vi "压电喷油器控制-与PLC进行串行通信完善喷油延时.vi"() -> ()   [LabVIEW 2018]
uses:
  <vilib>/Instr/_visa.llb/VISA Configure Serial Port (Instr).vi
panel:
  in  "充放电时间US":dbl[](array[numeric])=[30.0, 0.0, 70.0, 1.0, 50.0, 1.0, 0.0, 0.0, 0.0, 0.0, 0.0, 30.0]
  out "返回指令码":dbl[](array[numeric])
  in  "确定 3":bool
  in  "VISA资源名称 3":refnum<visa-resource-name>
  out "返回指令码":dbl[](array[numeric])
  in  "确定 2":bool
  in  "VISA资源名称 2":refnum<visa-resource-name>
  in  "喷油间隔设定  US":dbl[](array[numeric])=[20.0, 0.0, 0.0, 0.0, 0.0, 0.0, 0.0, 0.0, 0.0, 0.0, 0.0, 20.0]
  out "返回指令码":dbl[](array[numeric])
  in  "喷油脉宽设定 US":dbl[](array[numeric])=[10.0, 0.0, 0.0, 0.0, 0.0, 0.0, 0.0, 0.0, 0.0, 0.0, 0.0, 10.0]
  in  "允许通讯":bool
  in  "确定1":bool
  in  "VISA资源名称":refnum<visa-resource-name>
  # "每次打开上位机界面，有的数据表格可能不需要输入数据，如喷油4次，则第五个数据就不需要输入，但\n是仍然要向其写入0，相当于赋初值，否则报错。"
  # "注\n意"
  # "说明：每一行数据的第一个数据都表示指令码，其中喷油脉宽设定的指令码是10，因此第一个框中只能输入10，类似的，其余变量的指令码如下：\n喷油脉宽设定10，喷油间隔设定20，充放电时间及次数设定30"
  # "脉宽\n设定"
  # "末位校验，必须输入10"
  # "脉宽1（千百位）"
  # "脉宽1（十个位）"
  # "脉宽2（千百位）"
  # "脉宽2（十个位）"
  # "脉宽3（千百位）"
  # "脉宽3（十个位）"
  # "脉宽4（千百位）"
  # "脉宽5（千百位）"
  # "脉宽5（十个位）"
  # "脉宽4（十个位）"
  # "指令框：第一个只能\n输入10"
  # "间隔\n设定"
  # "间隔2（千百位）"
  # "间隔3（千百位）"
  # "间隔3（十个位）"
  # "末位校验，必须输入20"
  # "延时（十个位）"
  # "间隔2（十个位）"
  # "间隔1（十个位）"
  # "间隔4（十个位）"
  # "间隔1（千百位）"
  # "间隔4（千百位）"
  # "延时（千百位）"
  # "指令框：第一个只能\n输入20"
  # "间隔的万千位能够设置的最大值为65，即65ms"
  # "时间\n次数\n设定"
  # "充电时间\n（十个位）"
  # "放电时间\n（十个位）"
  # "充电时间\n（百位）"
  # "放电时间\n（百位）"
  # "喷油次数"
  # "不用"
  # "不用"
  # "不用"
  # "不用"
  # "不用"
  # "末位校验，必须输入30"
  # "指令框：第一个只能输入30"
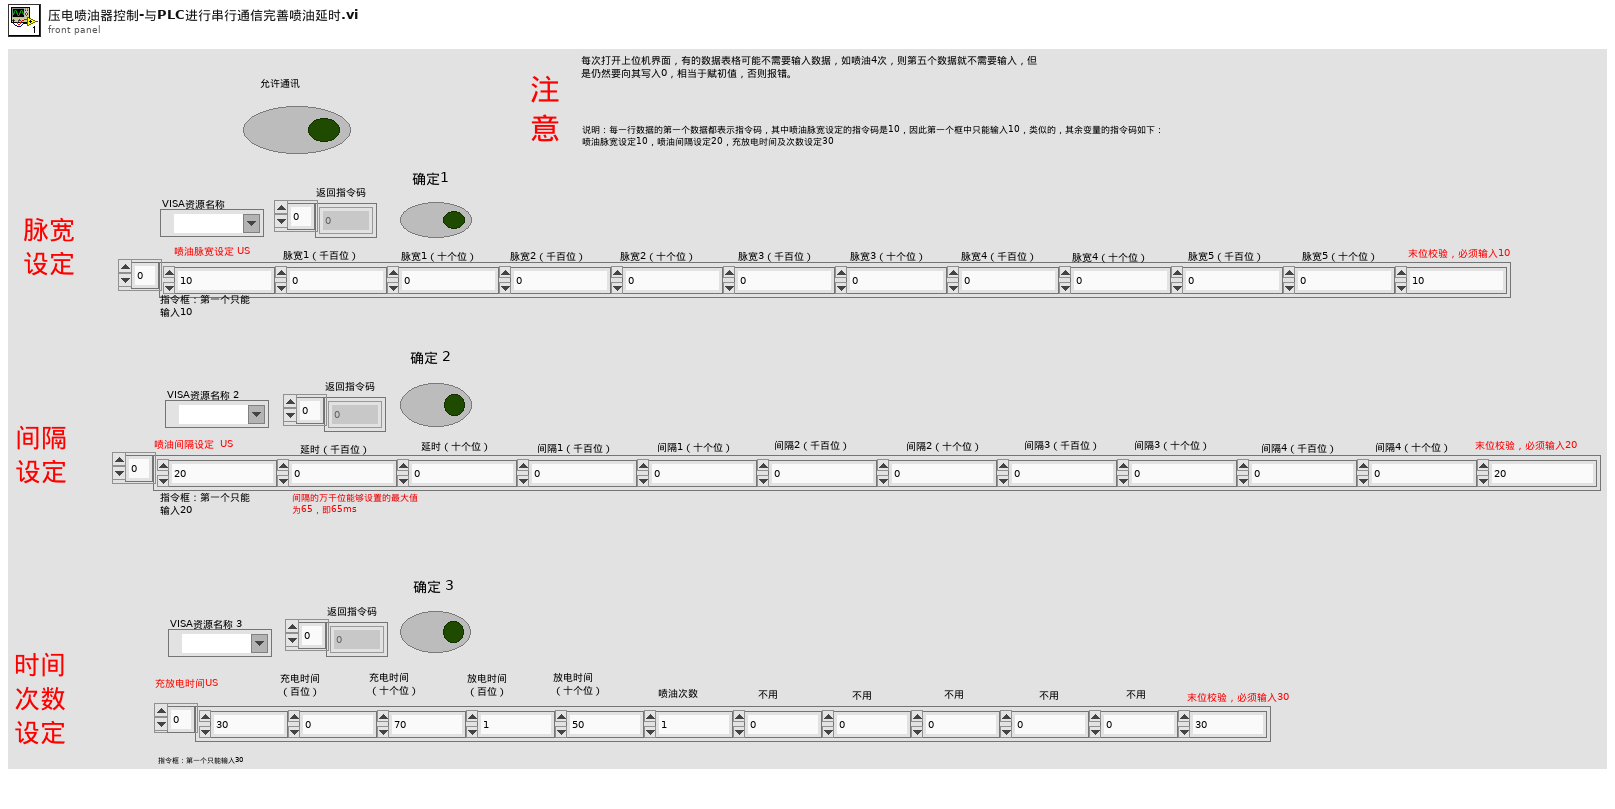
[diagram p1: front panel]
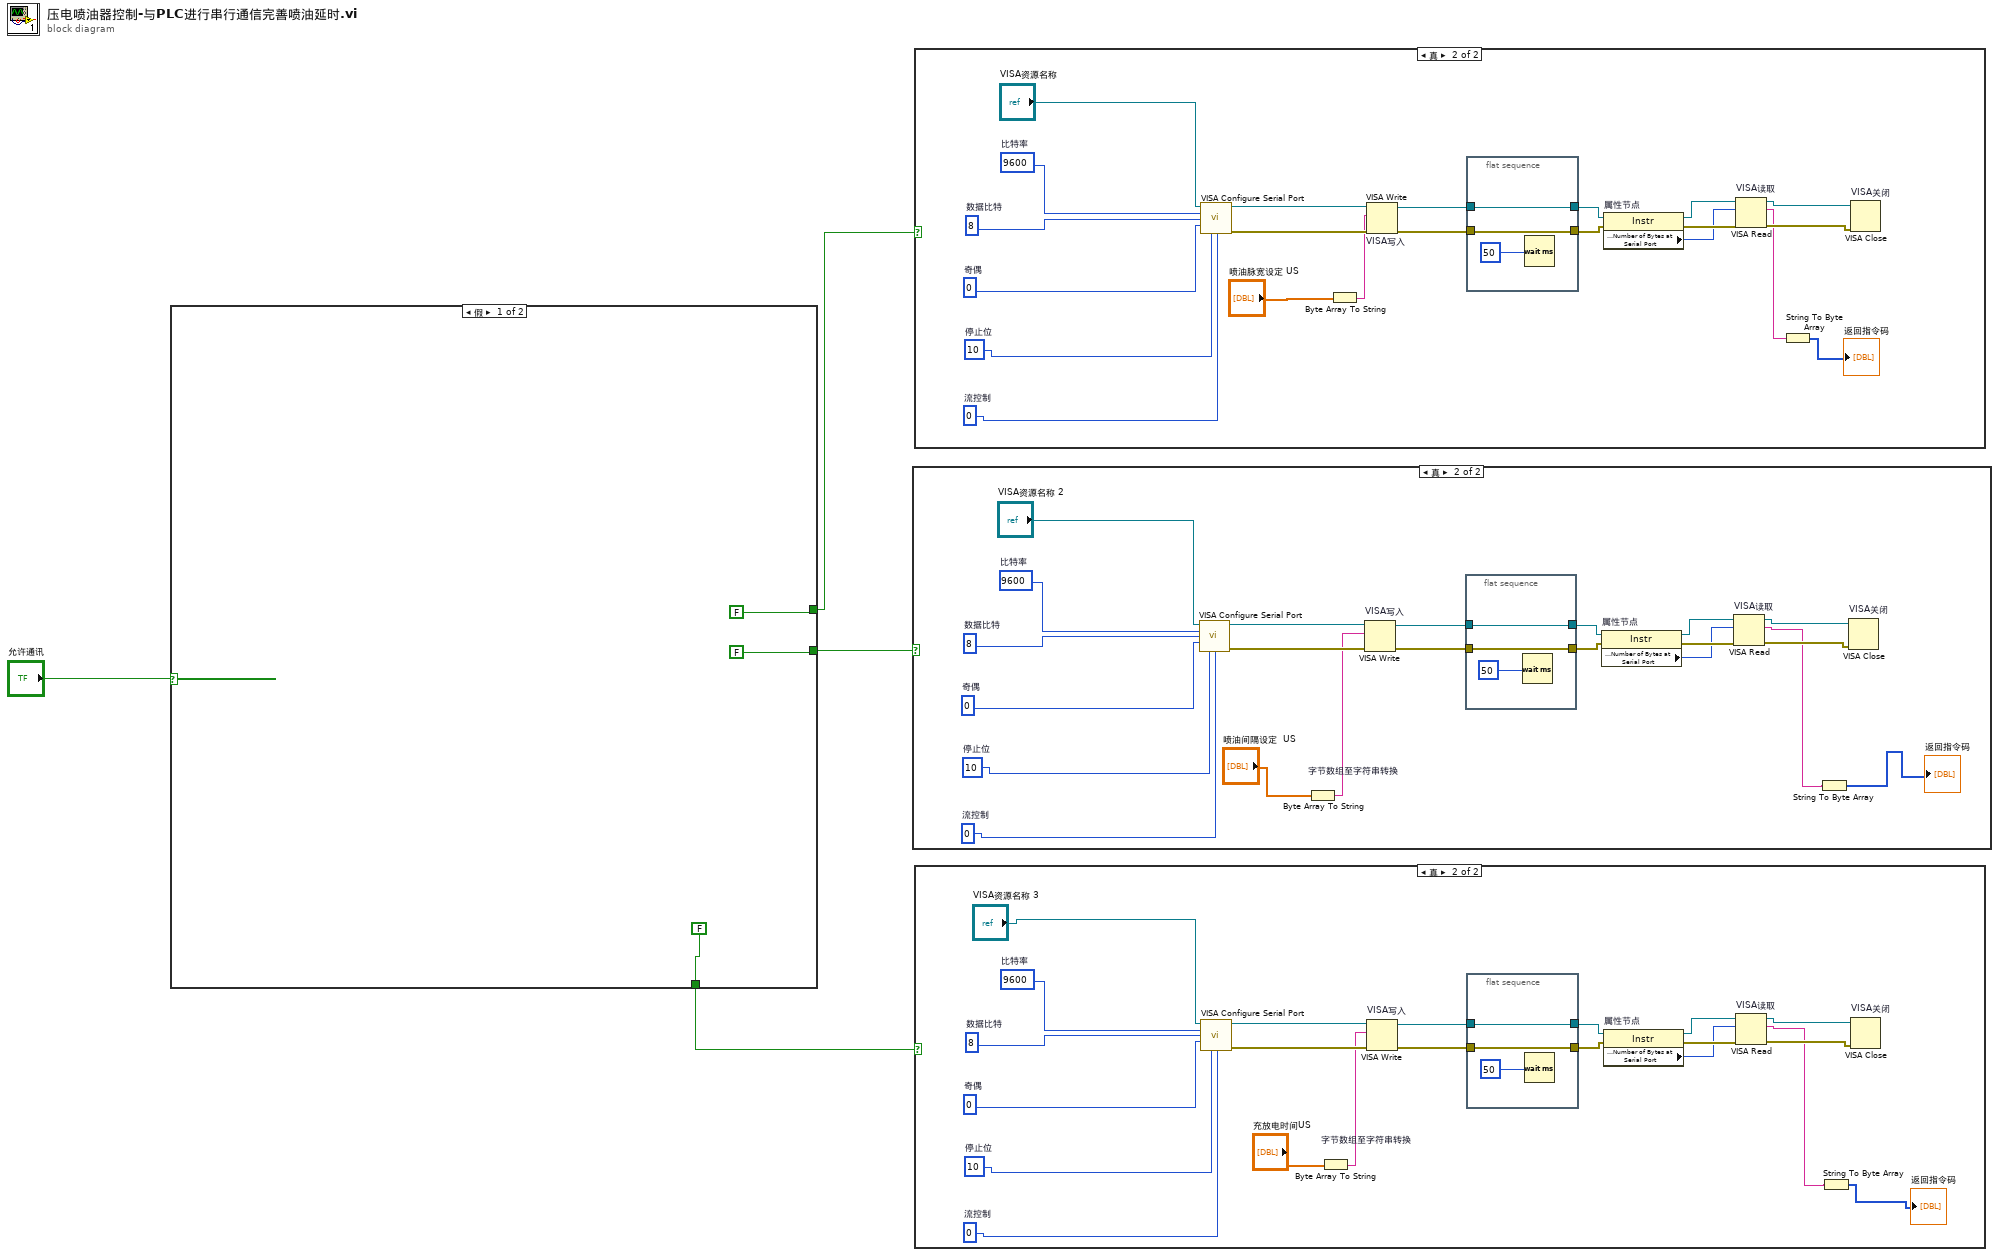
[diagram p0: block diagram]
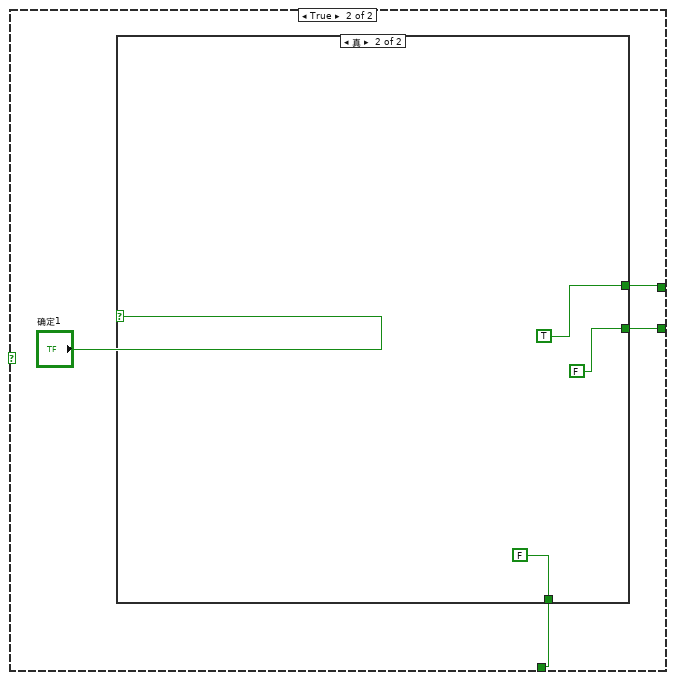
[diagram p2: hidden frame]
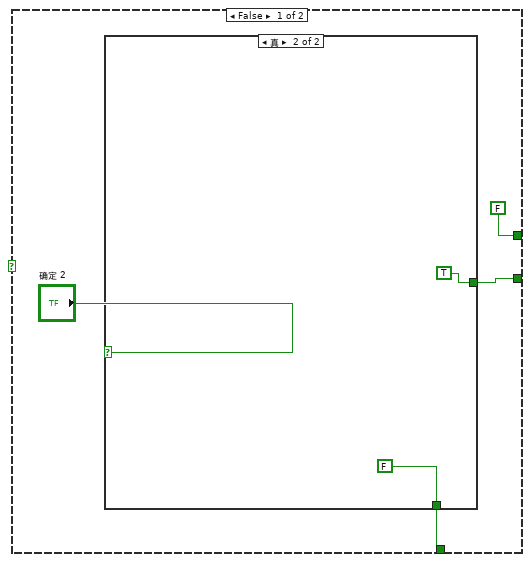
[diagram p3: hidden frame]
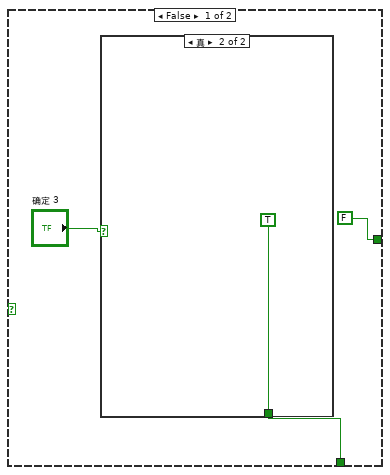
[diagram p4: hidden frame]
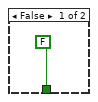
[diagram p5: hidden frame]
diagram:
  n1 = case shown="假" "允许通讯" {
    tunnel: [FALSE w10] -> w3
    tunnel: [FALSE w9] -> w2
    tunnel: [FALSE w8] -> w1
    frame False {
    }
    frame True {
      n2 = case shown="真" "确定1" {
        tunnel: [FALSE TRUE] -> w10
        tunnel: [w13 FALSE] -> w9
        tunnel: [w12 FALSE] -> w8
        frame False {
          n3 = case "条件结构" shown="真" "确定 2" {
            tunnel: [FALSE TRUE] -> w13
            tunnel: [w17 FALSE] -> w12
            frame False {
              n4 = case shown="真" "确定 3" {
                tunnel: [FALSE TRUE] -> w17
                frame False {
                }
                frame True {
                }
              }
            }
            frame True {
            }
          }
        }
        frame True {
        }
      }
    }
  }
  n5 = case shown="真" w2 {
    frame False {
    }
    frame True {
      w30 = 0  # 流控制
      w31 = 10  # 停止位
      w32 = 0  # 奇偶
      w33 = 8  # 数据比特
      w34 = 9600  # 比特率
      n6 = call-poly "VISA Configure Serial Port"("VISA resource name"="VISA资源名称 2", "baud rate (9600)"=w34, "data bits (8)"=w33, "parity (0:none)"=w32, "stop bits (10: 1 bit)"=w31, "flow control (0:none)"=w30) -> ("VISA resource name out"=w40:refnum<visa-resource-name>, "error out"=w39:errorcluster)  [unwired: 8 in]
      n7 = Byte Array To String "字节数组至字符串转换"(unsigned byte array="喷油间隔设定  US") -> (string=w29:string)
      n8 = VISA Write "VISA写入"(VISA resource name=w40, write buffer=w29, error in (no error)=w39) -> (VISA resource name out=w37:refnum<visa-resource-name>, error out=w35:errorcluster)  [unwired: 1 out]
      n9 = flat-sequence {
        tunnel: [w49] -> w38
        tunnel: w37 -> [w49]
        tunnel: [w48] -> w36
        tunnel: w35 -> [w48]
        frame #0 {
          n10 = Wait (ms)(milliseconds to wait=50) -> ()  [unwired: 1 out]
        }
      }
      n11 = property on="属性节点" class="Instr"(reference=w38, error in=w36) -> (reference out=w45:refnum<visa-resource-name>, error out=w44:errorcluster, "Serial Settings:Number of Bytes at Serial Port"=w41:u32)
      n12 = VISA Read "VISA读取"(VISA resource name=w45, byte count=w41, error in (no error)=w44) -> (VISA resource name out=w43:refnum<visa-resource-name>, read buffer=w26:string, error out=w42:errorcluster)  [unwired: 1 out]
      n13 = String To Byte Array(string=w26) -> (unsigned byte array=→"返回指令码":u8[])
      n14 = VISA Close "VISA关闭"(VISA resource name=w43, error in (no error)=w42) -> ()  [unwired: 1 out]
    }
  }
  n15 = case shown="真" w3 {
    frame False {
    }
    frame True {
      w54 = 0  # 流控制
      w55 = 10  # 停止位
      w56 = 0  # 奇偶
      w57 = 8  # 数据比特
      w58 = 9600  # 比特率
      n16 = call-poly "VISA Configure Serial Port"("VISA resource name"="VISA资源名称", "baud rate (9600)"=w58, "data bits (8)"=w57, "parity (0:none)"=w56, "stop bits (10: 1 bit)"=w55, "flow control (0:none)"=w54) -> ("VISA resource name out"=w64:refnum<visa-resource-name>, "error out"=w63:errorcluster)  [unwired: 8 in]
      n17 = Byte Array To String(unsigned byte array="喷油脉宽设定 US") -> (string=w53:string)
      n18 = VISA Write "VISA写入"(VISA resource name=w64, write buffer=w53, error in (no error)=w63) -> (VISA resource name out=w61:refnum<visa-resource-name>, error out=w59:errorcluster)  [unwired: 1 out]
      n19 = flat-sequence {
        tunnel: [w73] -> w62
        tunnel: w61 -> [w73]
        tunnel: [w72] -> w60
        tunnel: w59 -> [w72]
        frame #0 {
          n20 = Wait (ms)(milliseconds to wait=50) -> ()  [unwired: 1 out]
        }
      }
      n21 = property on="属性节点" class="Instr"(reference=w62, error in=w60) -> (reference out=w69:refnum<visa-resource-name>, error out=w68:errorcluster, "Serial Settings:Number of Bytes at Serial Port"=w65:u32)
      n22 = VISA Read "VISA读取"(VISA resource name=w69, byte count=w65, error in (no error)=w68) -> (VISA resource name out=w67:refnum<visa-resource-name>, read buffer=w50:string, error out=w66:errorcluster)  [unwired: 1 out]
      n23 = String To Byte Array(string=w50) -> (unsigned byte array=→"返回指令码":u8[])
      n24 = VISA Close "VISA关闭"(VISA resource name=w67, error in (no error)=w66) -> ()  [unwired: 1 out]
    }
  }
  n25 = case shown="真" w1 {
    frame False {
    }
    frame True {
      w79 = 0  # 流控制
      w80 = 10  # 停止位
      w81 = 0  # 奇偶
      w82 = 8  # 数据比特
      w83 = 9600  # 比特率
      n26 = call-poly "VISA Configure Serial Port"("VISA resource name"="VISA资源名称 3", "baud rate (9600)"=w83, "data bits (8)"=w82, "parity (0:none)"=w81, "stop bits (10: 1 bit)"=w80, "flow control (0:none)"=w79) -> ("VISA resource name out"=w89:refnum<visa-resource-name>, "error out"=w88:errorcluster)  [unwired: 8 in]
      n27 = Byte Array To String "字节数组至字符串转换"(unsigned byte array="充放电时间US") -> (string=w75:string)
      n28 = VISA Write "VISA写入"(VISA resource name=w89, write buffer=w75, error in (no error)=w88) -> (VISA resource name out=w86:refnum<visa-resource-name>, error out=w84:errorcluster)  [unwired: 1 out]
      n29 = flat-sequence {
        tunnel: [w97] -> w87
        tunnel: w86 -> [w97]
        tunnel: [w96] -> w85
        tunnel: w84 -> [w96]
        frame #0 {
          n30 = Wait (ms)(milliseconds to wait=50) -> ()  [unwired: 1 out]
        }
      }
      n31 = property on="属性节点" class="Instr"(reference=w87, error in=w85) -> (reference out=w94:refnum<visa-resource-name>, error out=w93:errorcluster, "Serial Settings:Number of Bytes at Serial Port"=w90:u32)
      n32 = VISA Read "VISA读取"(VISA resource name=w94, byte count=w90, error in (no error)=w93) -> (VISA resource name out=w92:refnum<visa-resource-name>, read buffer=w78:string, error out=w91:errorcluster)  [unwired: 1 out]
      n33 = String To Byte Array(string=w78) -> (unsigned byte array=→"返回指令码":u8[])
      n34 = VISA Close "VISA关闭"(VISA resource name=w92, error in (no error)=w91) -> ()  [unwired: 1 out]
    }
  }
